vi "Autonomous.vi"   [LabVIEW 2020]
doc: "This VI starts when autonomous period begins, and will automatically be terminated when it ends. You can carry out timed or sensor driven operations directly to I/O or to subsystems without needing to return to the caller."
uses:
  Framework/Robot Global Data.vi
  Drive/Implementation/Infrastructure/Drive Command Helper.vi
  <vilib>/Rock Robotics/WPI/ThirdParty/Phoenix-LabVIEW/Pigeon IMU/CTRE_PigeonIMU_GetYPR.vi
types:
  T1 = typedef "Single Cmd Info.ctl" = cluster{"Name":string, "CPTM.DataType":variant, "All Control Values Variant":cluster{"Name":string, "Variant Data":variant}[], "icon full":T2, "icon scaled":T2, "Path":path, "Subsystem Color":u32}
  T2 = typedef "imagedata.ctl" = cluster{"image type":i32, "image depth":i32, "image":u8[], "mask":u8[], "colors":u32[], "Rectangle":cluster{"left":i16, "top":i16, "right":i16, "bottom":i16}}
  T3 = typedef "Trajectory Data.ctl" = cluster{"Segment Name":string, "Type":T4, "Traj Pos Points":cluster{"x":dbl, "y":dbl, "th":dbl}[], "Traj Vel Points":cluster{"V":dbl, "Omega":dbl, "V vector":cluster{"y":dbl, "x":dbl}}[], "Accel Index":i32, "Decel Index":i32}[]
  T4 = typedef "Segment Type.ctl" = enum16{"Accel Straight", "Const Straight", "Blend", "Circle", "Bezier"}
  T5 = typedef "Overrides.ctl" = cluster{"Count":string, "Angular Override":dbl, "Enabled?":bool, "Velocity Override":dbl, "Angle Override":dbl}[]
  T6 = typedef "Angluar Limits.ctl" = cluster{"Velocity (deg/s)":dbl, "Accel (deg/s^2)":dbl, "Jerk (deg/s^3)":dbl}
  T7 = typedef "Drive Type.ctl" = enum16{"Nonholonomic", "Holonomic"}
  T8 = typedef "Path Type.ctl" = enum16{"Clothoid", "Bezier"}
  T9 = cluster{"Overall":cluster{"Time (s)":dbl, "Distance (ft)":dbl}, "Points out":cluster{"x":dbl, "y":dbl, "th":dbl}[], "Commands out":cluster{"Time (s)":dbl, T1, bool}[], "Zero V":bool, "Trajectory Data":T3, "Reversals":cluster{"Robot Backwards":bool, "Reverse Path":bool}, "Fields":cluster{"Sample Period (s)":dbl, cluster{"Velocity (fps)":dbl, "Accel (fps^2)":dbl, "Jerk (fps^3)":dbl, "StoopidFast (fps)":dbl}, "Conditions":cluster{"vInitial (fps)":dbl, "vFinal (fps)":dbl}, "Overrides":T5, "Angular Limits":T6}, "Trajectory Meta":cluster{"Drive Type":T7, "Path Type":T8}}[]
  T10 = cluster{"Robot Backwards":bool, "Reverse Path":bool}
  T11 = cluster{"V":dbl, "Omega":dbl, "V vector":cluster{"y":dbl, "x":dbl}}[]
  T12 = cluster{"Segment Name":string, "Type":T4, "Traj Pos Points":cluster{"x":dbl, "y":dbl, "th":dbl}[], "Traj Vel Points":cluster{"V":dbl, "Omega":dbl, "V vector":cluster{"y":dbl, "x":dbl}}[], "Accel Index":i32, "Decel Index":i32}
  T13 = cluster{cluster{"y":dbl, "x":dbl}[], cluster{dbl, dbl}[], cluster{"Time (s)":dbl, T1, bool}[], i32[]}
  T14 = typedef "CTRE_PigeonIMU_DeviceRef.ctl" = cluster{"DeviceStatus":errorcluster, "Device Number":u8, "Type":T15, "Device ID":u32, "Handle":u64, "UsageFrame":u32, "Library Path":path}
  T15 = typedef "CTRE_PigeonIMU_ConnectionType.ctl" = u32
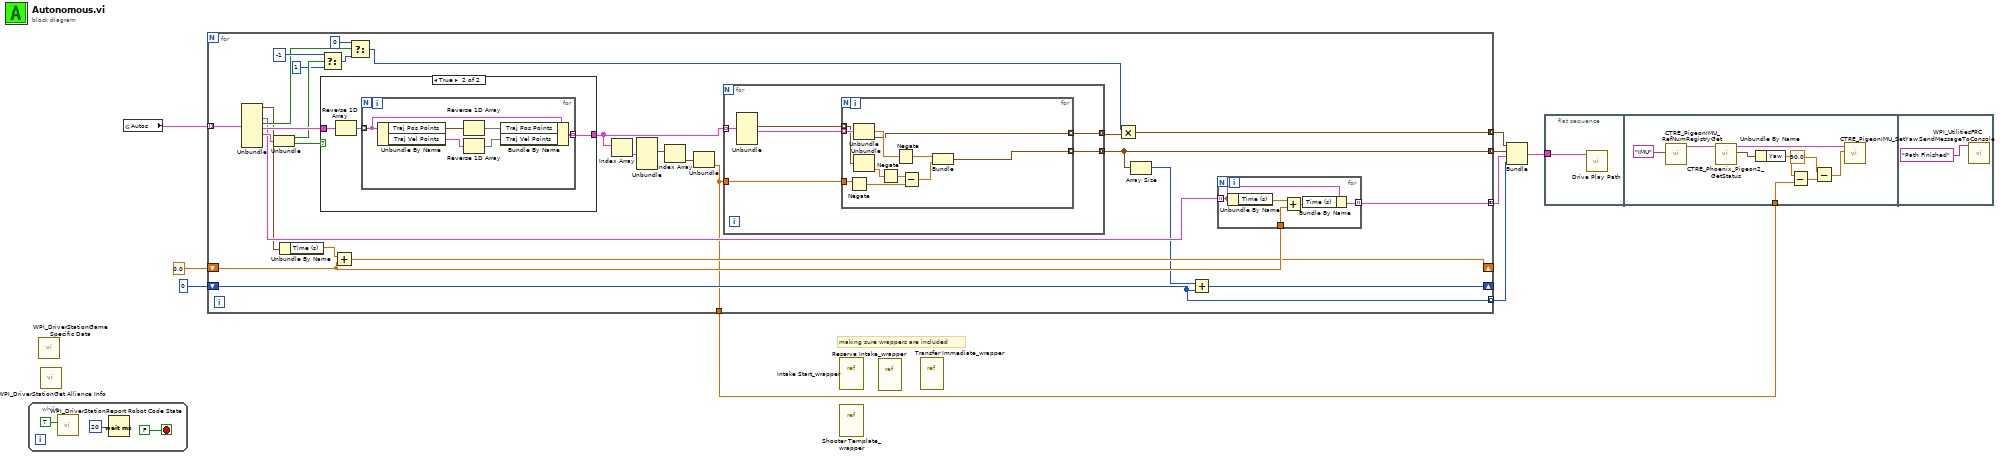
[diagram p0: block diagram]
diagram:
  # "making sure wrappers are included"
  n1 = while {
    stop <- FALSE stop-if-true
    n2 = call <vilib>:"WPI_DriverStationReport Robot Code State.vi"("Autonomous"=TRUE) -> ()  [unwired: 10 in, 1 out]
    n3 = Wait (ms)(milliseconds to wait=u32 20) -> ()  [unwired: 1 out]
  }
  n4 = call <vilib>:"WPI_DriverStationGame Specific Data.vi"() -> ()  [unwired: 11 in, 1 out]
  n5 = call <vilib>:"WPI_DriverStationGet Alliance Info.vi"() -> ()  [unwired: 12 out]
  n6 = global read "Robot Global Data.vi" "Autos"() -> (w9:T9)
  n7 = for {
    tunnel: w9 -> [w40] mode=indexing
    shift-right: [w19] -> _
    shift-left: 0.0 -> [w20]
    tunnel: [w24] -> w7 mode=concatenating
    tunnel: [w17] -> w6 mode=concatenating
    tunnel: [w18] -> w5 mode=concatenating
    shift-right: [w15] -> _
    shift-left: 0 -> [w14]
    tunnel: [w14] -> w2 mode=indexing
    tunnel: [w13] -> w1
    n8 = Unbundle(w40) -> ("Overall"=w22:cluster{"Time (s)":dbl, "Distance (ft)":dbl}, "Commands out"=w23:cluster{"Time (s)":dbl, T1, bool}[], "Zero V"=w26:bool, "Trajectory Data"=w38:T3, "Reversals"=w39:T10)  [unwired: 3 out]
    n9 = Unbundle(w39) -> ("Robot Backwards"=w36:bool, "Reverse Path"=w37:bool)
    n10 = Unbundle By Name(w22) -> ("Time (s)"=w21:dbl)
    n11 = case shown="True" w37 {
      tunnel: w38 -> [w63 w66]
      tunnel: [w63 w64] -> w32
      frame False {
      }
      frame True {
        n12 = Reverse 1D Array(array=w66) -> (reversed array=w65:T3)
        n13 = for {
          tunnel: w65 -> [w72] mode=indexing
          tunnel: [w67] -> w64 mode=indexing
          n14 = Unbundle By Name(w72) -> ("Traj Pos Points"=w71:cluster{"x":dbl, "y":dbl, "th":dbl}[], "Traj Vel Points"=w69:T11)
          n15 = Reverse 1D Array(array=w71) -> (reversed array=w70:cluster{"x":dbl, "y":dbl, "th":dbl}[])
          n16 = Reverse 1D Array(array=w69) -> (reversed array=w68:T11)
          n17 = Bundle By Name(cluster=w72, "Traj Pos Points"=w70, "Traj Vel Points"=w68) -> (w67:T12)
        }
      }
    }
    n18 = Select(t=-1, s=w36, f=1) -> (s? t:f=w28:i32)
    n19 = Add(x=w21, y=w20) -> (x+y=w19:dbl)
    n20 = Select(t=0, s=w26, f=w28) -> (s? t:f=w25:i32)
    n21 = Index Array(array=w32) -> (element=w31:T12)  [unwired: 1 in]
    n22 = Unbundle(w31) -> ("Traj Pos Points"=w30:cluster{"x":dbl, "y":dbl, "th":dbl}[])  [unwired: 5 out]
    n23 = Index Array(array=w30) -> (element=w29:cluster{"x":dbl, "y":dbl, "th":dbl})  [unwired: 1 in]
    n24 = Unbundle(w29) -> ("th"=w13:dbl)  [unwired: 2 out]
    n25 = for {
      tunnel: w32 -> [w51] mode=indexing
      tunnel: [w50] -> w33 mode=concatenating
      tunnel: [w49] -> w17 mode=concatenating
      tunnel: w13 -> [w46]
      # "/shrug"
      n26 = Unbundle(w51) -> ("Traj Pos Points"=w47:cluster{"x":dbl, "y":dbl, "th":dbl}[], "Traj Vel Points"=w48:T11)  [unwired: 4 out]
      n27 = for {
        tunnel: w48 -> [w62] mode=indexing
        tunnel: [w52] -> w50 mode=indexing
        tunnel: [w61] -> w49 mode=indexing
        tunnel: w47 -> [w60] mode=indexing
        tunnel: w46 -> [w57]
        n28 = Negate(x=w57) -> (-x=w53:dbl)
        n29 = Unbundle(w62) -> ("Omega"=w58:dbl, "V vector"=w52:cluster{"y":dbl, "x":dbl})  [unwired: 1 out]
        n30 = Unbundle(w60) -> ("th"=w56:dbl)  [unwired: 2 out]
        n31 = Negate(x=w56) -> (-x=w54:dbl)
        n32 = Negate(x=w58) -> (-x=w55:dbl)
        n33 = Subtract(x=w54, y=w53) -> (x-y=w59:dbl)
        n34 = Bundle(w55, w59) -> (w61:cluster{dbl, dbl})  [unwired: 1 in]
      }
    }
    n35 = Multiply(x=w25, y=w33) -> (x*y=w24:cluster{"y":dbl, "x":dbl}[])
    n36 = Array Size(array=w17) -> (size(s)=w16:i32)
    n37 = Add(x=w16, y=w14) -> (x+y=w15:i32)
    n38 = for {
      tunnel: w23 -> [w42] mode=indexing
      tunnel: w20 -> [w44]
      tunnel: [w41] -> w18 mode=indexing
      n39 = Unbundle By Name(w42) -> ("Time (s)"=w45:dbl)
      n40 = Add(x=w45, y=w44) -> (x+y=w43:dbl)
      n41 = Bundle By Name(cluster=w42, "Time (s)"=w43) -> (w41:cluster{"Time (s)":dbl, T1, bool})
    }
  }
  n42 = vi-ref "Intake Start_wrapper.vi"() -> ()  [unwired: 1 out]
  n43 = vi-ref "Shooter Template_wrapper.vi"() -> ()  [unwired: 1 out]
  n44 = vi-ref "Reserve Intake_wrapper.vi"() -> ()  [unwired: 1 out]
  n45 = vi-ref "Transfer Immediate_wrapper.vi"() -> ()  [unwired: 1 out]
  n46 = Bundle(w7, w6, w5, w2) -> (w4:T13)  [unwired: 1 in]
  n47 = flat-sequence {
    tunnel: w4 -> [w73]
    tunnel: w1 -> [w77]
    frame #0 {
      n48 = call "Drive Play Path.vi"("Swerve Path Data"=w73) -> ()  [unwired: 10 in, 1 out]
    }
    frame #1 {
      n49 = call <vilib>:"CTRE_PigeonIMU_RefNumRegistryGet.vi"("refnum name"="IMU") -> ("PigeonIMUDevRef"=w81:T14)  [unwired: 9 in, 1 out]
      n50 = call-poly <vilib>:"CTRE_Phoenix_Pigeon2_GetStatus.vi"("PigeonIMUDevRef"=w81) -> ("Yaw Pitch Roll"=w80:cluster{"Yaw":dbl, "Pitch":dbl, "Roll":dbl}, "PigeonIMUDevRef"=w79:T14)  [unwired: 8 in, 1 out]
      n51 = Unbundle By Name(w80) -> ("Yaw"=w78:dbl)
      n52 = Subtract(x=w78, y=w77) -> (x-y=w76:dbl)
      n53 = Subtract(x=90.0, y=w76) -> (x-y=w74:dbl)
      n54 = call <vilib>:"CTRE_PigeonIMU_SetYaw.vi"("Value"=w74, "PigeonIMUDevRef"=w79) -> ()  [unwired: 8 in, 2 out]
    }
    frame #2 {
      n55 = call <vilib>:"WPI_UtilitiesFRC SendMessageToConsole.vi"("Message"="Path Finished") -> ()  [unwired: 14 in, 1 out]
    }
  }
